vi "FPGA Write.vi"(8 "error in":errorcluster, 11 "FPGA VI Reference In":refnum<k20>) -> (0 "error out":errorcluster, 3 "FPGA VI Reference Out":refnum<k20>)   [LabVIEW 2011]
uses:
  <vilib>/Utility/error.llb/Error Cluster From Error Code.vi
  <vilib>/rvi/errors/niLvFpgaAdjustHostInterfaceError.vi
  <vilib>/rvi/interface/nirviReadWriteControl/nirviReadWriteControl.xnode
  NiFpgaLv.dll
  <vilib>/rvi/interface/Simulation/niFpgaSimulationCallBeginRW.vi
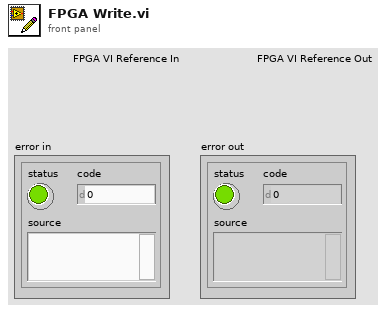
[diagram p1: front panel]
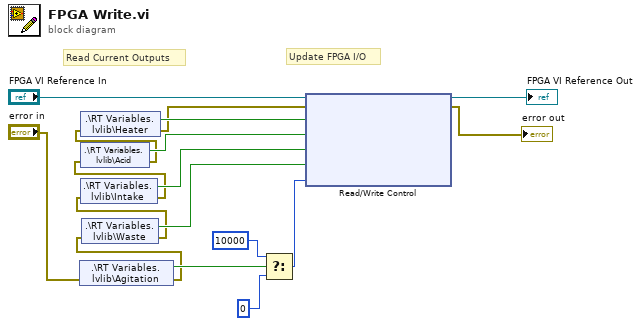
[diagram p0: block diagram]
diagram:
  # "Update FPGA I/O"
  # "Read Current Outputs"
  n1 = shared-variable ".\\RT Variables.lvlib\\Agitation"(error in="error in") -> (w11:bool, error out=w6:errorcluster)
  n2 = shared-variable ".\\RT Variables.lvlib\\Waste"(error in=w6) -> (w12:bool, error out=w5:errorcluster)
  n3 = shared-variable ".\\RT Variables.lvlib\\Intake"(error in=w5) -> (w13:bool, error out=w4:errorcluster)
  n4 = shared-variable ".\\RT Variables.lvlib\\Acid"(error in=w4) -> (w14:bool, error out=w3:errorcluster)
  n5 = shared-variable ".\\RT Variables.lvlib\\Heater"(error in=w3) -> (w15:bool, error out=w2:errorcluster)
  n6 = Select(t=10000, s=w11, f=0 ("PWM Duty Cycle (Ticks)")) -> (s? t:f=w8:i32)
  n7 = xnode "Read/Write Control"("FPGA VI Reference In"="FPGA VI Reference In", "error in"=w2, "Heater"=w15, "Acid"=w14, "Intake"=w13, "Waste"=w12, "PWM Duty Cycle (Ticks)"=w8) -> ("FPGA VI Reference Out"=→"FPGA VI Reference Out":refnum<k20>, "error out"=→"error out":errorcluster)
